vi "Delete Scale.vi"(8 "error in (no error)":errorcluster, 10 "Index":i32, 11 "references":T1) -> (0 "error out":errorcluster)   [LabVIEW 2014, in "Scaling editor node.lvclass"]
uses:
  Scaling editor node.lvclass
  <vilib>/NI/DCAF/Tag Editor Core/Table API/Table Manager/object ref.ctl
  <vilib>/NI/DCAF/Tag Editor Core/Configuration Editor/Classes/Engine Parent/Engine Parent Editor Node.lvclass
  <vilib>/NI/DCAF/Tag Editor Core/Configuration Editor/Classes/Module editor node/module editor node.lvclass
  module/configuration/Scaling configuration.lvclass
  <vilib>/NI/Configuration Framework/serializable configuration/NISE_CEF_serializable configuration.lvclass/NISE_CEF_serializable configuration.ctl
  <vilib>/Utility/LVClass/Get LV Class Name.vi
  <vilib>/NI/Configuration Framework/error generator/NISE_error generator.vi
  <vilib>/NI/Configuration Framework/serializable configuration/NISE_CEF_serializable configuration.lvclass
  <vilib>/NI/Module Execution Interface/Engine Configuration/engine configuration.lvclass
  <vilib>/NI/DCAF/Tag Editor Core/Table API/Table Manager/Table Manager.lvclass
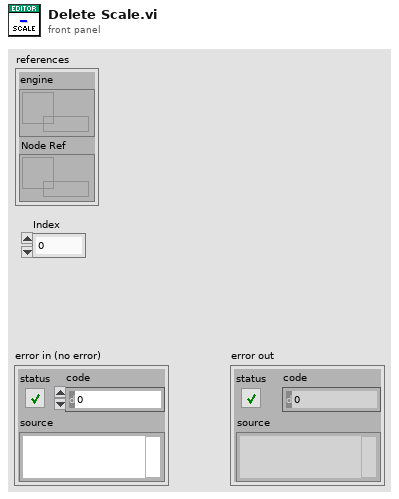
[diagram p1: front panel]
types:
  T1 = typedef "Table Manager.lvlib/Table Manager.lvclass/object ref.ctl" = cluster{"engine":refnum<data-value>, "Node Ref":refnum<data-value>}
  T2 = typedef "Scaling configuration.lvclass/scale data types.ctl" = enum16{"Double", "Single", "I64", "I32", "I16", "I8", "U64", "U32", "U16", "U8", "Boolean"}
  T3 = cluster{"mappings":cluster{"input channel":refnum<class "TBM channel.lvclass">, "output channel":refnum<class "TBM channel.lvclass">, "input data type":T2, "output data type":T2}[], "name":string}
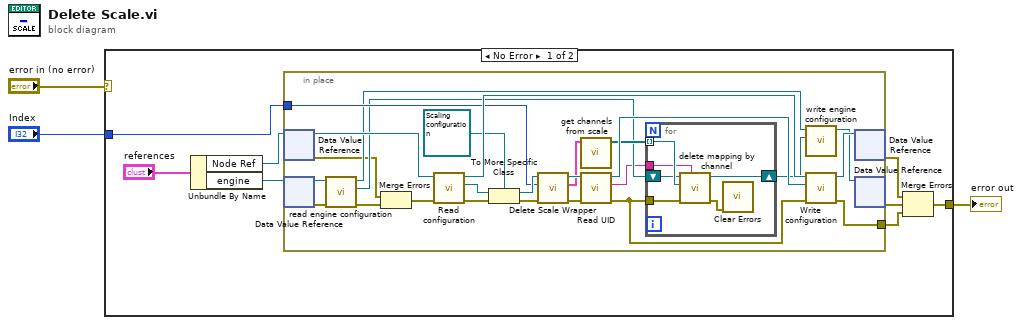
[diagram p0: block diagram]
diagram:
  n1 = case shown="No Error" "error in (no error)" {
    selector: "error in (no error)" -> [_ w44]
    tunnel: [w4 w44] -> w1
    tunnel: "Index" -> [w9 _]
    frame No Error {
      n2 = Unbundle By Name("references") -> ("Node Ref"=w10:refnum<data-value>, "engine"=w8:refnum<data-value>)
      n3 = in-place {
        in-place-border: [w33] -> w5
        in-place-border: w9 -> [w28]
        n4 = in-place-dvr #1(w10) -> (w36:refnum<class "module editor node.lvclass">, w16:errorcluster)
        n5 = in-place-dvr #2(w8) -> (w27:refnum<class "Engine Parent Editor Node.lvclass">, w17:errorcluster)
        n6 = call <vilib>:"read engine configuration.vi"("error in"=w17, "Engine Parent Editor Node in"=w27) -> ("error out"=w15:errorcluster, "engine configuration"=w21:refnum<class "engine configuration.lvclass">, "Engine Parent Editor Node out"=w18:refnum<class "Engine Parent Editor Node.lvclass">)  [unwired: 7 in]
        n7 = Merge Errors(w16, w15) -> (w14:errorcluster)
        n8 = call-dynamic "Read configuration.vi"("error in"=w14, "NISE_CEF_serializable node in"=w36) -> ("error out"=w31:errorcluster, "configuration"=w35:refnum<class "NISE_CEF_serializable configuration.lvclass">, "NISE_CEF_serializable node out"=w37:refnum<class "module editor node.lvclass">)  [unwired: 7 in]
        n9 = To More Specific Class(target class=refnum<class "Scaling configuration.lvclass"> refnum ("Scaling configuration"), reference=w35, error in=w31) -> (specific class reference=w30:refnum<class "Scaling configuration.lvclass">, error out=w29:errorcluster)
        n10 = call "Delete Scale Wrapper.vi"("error in (no error)"=w29, "index"=w28, "Scaling configuration in"=w30) -> ("error out"=w24:errorcluster, "Deleted Scale"=w12:T3, "Scaling configuration out"=w25:refnum<class "Scaling configuration.lvclass">)  [unwired: 6 in]
        n11 = call "get channels from scale.vi"("Scale in"=w12) -> ("Channels"=w22:refnum<class "TBM channel.lvclass">[])  [unwired: 10 in]
        n12 = call <vilib>:"Read UID.vi"("error in"=w24, "configuration in"=w25) -> ("error out"=w13:errorcluster, "instance id"=w19:string, "configuration out"=w23:refnum<class "Scaling configuration.lvclass">)  [unwired: 7 in]
        n13 = for {
          tunnel: w22 -> [w43] mode=indexing
          shift-right: [w40] -> w20
          shift-left: w21 -> [w41]
          tunnel: w19 -> [w39]
          tunnel: w13 -> [w42]
          n14 = call <vilib>:"delete mapping by channel.vi"("owner ID"=w39, "error in"=w42, "channel"=w43, "engine configuration in"=w41) -> ("error out"=w38:errorcluster, "engine configuration out"=w40:refnum<class "engine configuration.lvclass">)  [unwired: 6 in]
          n15 = call <vilib>:"Clear Errors.vi"("error in (no error)"=w38) -> ()  [unwired: 5 in, 2 out]
        }
        n16 = call <vilib>:"write engine configuration.vi"("engine configuration"=w20, "Engine Parent Editor Node in"=w18) -> ("Engine Parent Editor Node out"=w26:refnum<class "Engine Parent Editor Node.lvclass">)  [unwired: 8 in, 1 out]
        n17 = call-dynamic "Write configuration.vi"("error in"=w13, "configuration"=w23, "NISE_CEF_serializable node in"=w37) -> ("error out"=w33:errorcluster, "NISE_CEF_serializable node out"=w34:refnum<class "module editor node.lvclass">)  [unwired: 7 in]
        n18 = in-place-dvr #1(w34) -> (w7:errorcluster)  [unwired: 1 out]
        n19 = in-place-dvr #2(w26) -> (w6:errorcluster)  [unwired: 1 out]
      }
      n20 = Merge Errors(w7, w6, w5) -> (w4:errorcluster)
    }
    frame Error {
    }
  }
  "error out" <- w1
